vi "InsertPts.vi"(1 "Array in":dbl[](array[numeric]) format="%.2f", 2 "pts to insert":u8=1) -> (0 "Array ouput":dbl[](array[numeric]) format="%.2f")   [LabVIEW 2022 SP3]
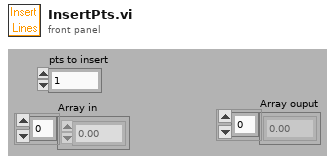
[diagram p1: front panel]
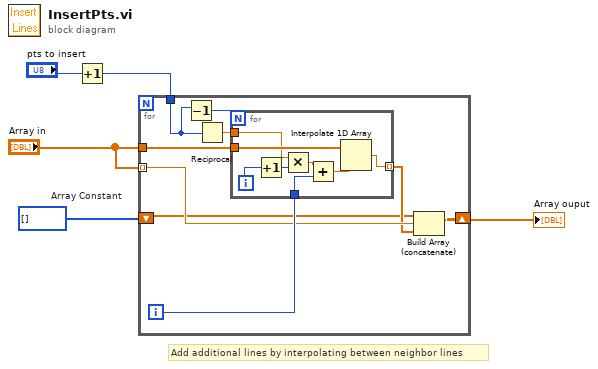
[diagram p0: block diagram]
diagram:
  w4 = i16[] []  # Array Constant
  # "Add additional lines by interpolating between neighbor lines"
  n1 = Increment(x="pts to insert") -> (x+1=w3:u8)
  n2 = for {
    tunnel: "Array in" -> [w12]
    tunnel: "Array in" -> [w11] mode=indexing
    shift-right: [w9] -> w1
    shift-left: w4 -> [w8]
    tunnel: w3 -> [w7]
    i -> [w14]
    n3 = Decrement(x=w7) -> (x-1=w6:u8)
    n4 = Reciprocal(x=w7) -> (1/x=w13:dbl)
    n5 = for {
      N: w6 -> [_]
      tunnel: w14 -> [w17]
      tunnel: w13 -> [w18]
      tunnel: w12 -> [w22]
      tunnel: [w21] -> w10 mode=indexing
      i -> [w20]
      n6 = Increment(x=w20) -> (x+1=w19:i32)
      n7 = Multiply(x=w18, y=w19) -> (x*y=w16:dbl)
      n8 = Add(x=w16, y=w17) -> (x+y=w15:dbl)
      n9 = Interpolate 1D Array(1:w15, 2:w22) -> (0:w21:dbl)
    }
    n10 = Build Array (concatenate)(w8, w11, w10) -> (w9:dbl[])
  }
  "Array ouput" <- w1
